vi "BoxBegin.vi"   [LabVIEW 2023]
uses:
  <vilib>/Rock Robotics/WPI/ThirdParty/REV Robotics/REVLib/Typedef/Spark MAX Idle Mode.ctl
  <vilib>/Rock Robotics/WPI/ThirdParty/REV Robotics/REVLib/Typedef/Spark MAX Sensor Type.ctl
  <vilib>/Rock Robotics/WPI/ThirdParty/REV Robotics/REVLib/Typedef/Spark MAX Motor Type.ctl
types:
  T1 = typedef "Spark MAX Sensor Type.ctl" = enum16{"No Sensor", "Hall Sensor", "Encoder", "-Not Available-", "Analog", "Alternate Encoder", "Duty Cycle"}
  T2 = typedef "Spark MAX Idle Mode.ctl" = enum16{"Coast", "Brake"}
  T3 = typedef "Spark MAX Motor Type.ctl" = enum16{"Brushed", "Brushless"}
  T4 = typedef "WPI_MotorControlDeviceRef.ctl" = cluster{"DeviceStatus":errorcluster, "Type":T5, "PWM":cluster{"PWM Channel":T6, "DeadBand":T7}, "CAN":cluster{"Device Number":u8, "SetOutput VI Ref":variant, "GetOutput VI Ref":variant, "Enable VI Ref":variant, "Disable VI Ref":variant, "Data":variant}, "Invert":bool, "DIO PWM":cluster{"PWM \"Enable\" Channel":T6, "DIOChannel":T8, "PWM Rate":dbl}}
  T5 = typedef "WPI_MotorControlType.ctl" = enum16{"PWM", "CAN", "DIO PWM"}
  T6 = typedef "FPGA_DIOPWMChannel.ctl" = enum8{"PWM 0", "PWM 1", "PWM 2", "PWM 3", "PWM 4", "PWM 5", "PWM 6", "PWM 7", "PWM 8", "PWM 9", "PWM MXP 0", "PWM MXP 1", "PWM MXP 2", "PWM MXP 3", "PWM MXP 4", "PWM MXP 5", "PWM MXP 6", "PWM MXP 7", "PWM MXP 8", "PWM MXP 9", "Invalid"}
  T7 = typedef "WPI_PWMDeadband.ctl" = cluster{"Name":string, "maxPositivePwm":i32, "minPositivePwm":i32, "centerPwm":i32, "maxNegativePwm":i32, "minNegativePwm":i32, "angularRange":u16}
  T8 = typedef "FPGA_DIOChannel.ctl" = enum8{"DIO 0", "DIO 1", "DIO 2", "DIO 3", "DIO 4", "DIO 5", "DIO 6", "DIO 7", "DIO 8", "DIO 9", "DIO MXP 0", "DIO MXP 1", "DIO MXP 2", "DIO MXP 3", "DIO MXP 4", "DIO MXP 5", "DIO MXP 6", "DIO MXP 7", "DIO MXP 8", "DIO MXP 9", "DIO MXP 10", "DIO MXP 11", "DIO MXP 12", "DIO MXP 13", "DIO MXP 14", "DIO MXP 15", "SPI Port CS1", "SPI Port CS2", "SPI Port CS3", "SPI Port MISO", "SPI Port MOSI", "Invalid"}
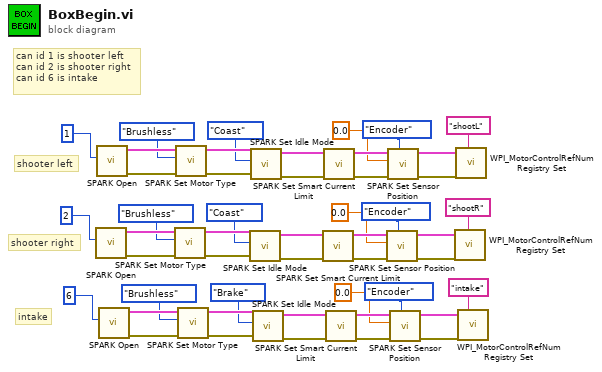
[diagram p0: block diagram]
diagram:
  # "intake"
  # "shooter right"
  # "shooter left"
  # "can id 1 is shooter left\ncan id 2 is shooter right\ncan id 6 is intake"
  n1 = call <vilib>:"SPARK Open.vi"("Device Number"=2) -> ("error out"=w25:errorcluster, "MotorControlDeviceRef"=w29:T4)  [unwired: 9 in]
  n2 = call <vilib>:"SPARK Open.vi"("Device Number"=1) -> ("error out"=w41:errorcluster, "MotorControlDeviceRef"=w45:T4)  [unwired: 9 in]
  n3 = call <vilib>:"SPARK Open.vi"("Device Number"=6) -> ("error out"=w9:errorcluster, "MotorControlDeviceRef"=w13:T4)  [unwired: 9 in]
  n4 = call <vilib>:"SPARK Set Motor Type.vi"("error in (no error)"=w25, "Motor Type"=Spark_MAX_Motor_Type."Brushless", "MotorControlDevRef"=w29) -> ("error out"=w24:errorcluster, "MotorControlDeviceRef"=w28:T4)  [unwired: 7 in]
  n5 = call <vilib>:"SPARK Set Motor Type.vi"("error in (no error)"=w41, "Motor Type"=Spark_MAX_Motor_Type."Brushless", "MotorControlDevRef"=w45) -> ("error out"=w40:errorcluster, "MotorControlDeviceRef"=w44:T4)  [unwired: 7 in]
  n6 = call <vilib>:"SPARK Set Motor Type.vi"("error in (no error)"=w9, "Motor Type"=Spark_MAX_Motor_Type."Brushless", "MotorControlDevRef"=w13) -> ("error out"=w8:errorcluster, "MotorControlDeviceRef"=w12:T4)  [unwired: 7 in]
  n7 = call <vilib>:"SPARK Set Idle Mode.vi"("error in (no error)"=w24, "Idle Mode"=Spark_MAX_Idle_Mode."Coast", "MotorControlDeviceRef in"=w28) -> ("error out"=w23:errorcluster, "MotorControlDeviceRef out"=w27:T4)  [unwired: 7 in]
  n8 = call <vilib>:"SPARK Set Idle Mode.vi"("error in (no error)"=w40, "Idle Mode"=Spark_MAX_Idle_Mode."Coast", "MotorControlDeviceRef in"=w44) -> ("error out"=w39:errorcluster, "MotorControlDeviceRef out"=w43:T4)  [unwired: 7 in]
  n9 = call <vilib>:"SPARK Set Idle Mode.vi"("error in (no error)"=w8, "Idle Mode"=Spark_MAX_Idle_Mode."Brake", "MotorControlDeviceRef in"=w12) -> ("error out"=w7:errorcluster, "MotorControlDeviceRef out"=w11:T4)  [unwired: 7 in]
  n10 = call <vilib>:"SPARK Set Smart Current Limit.vi"("error in (no error)"=w23, "MotorControlDeviceRef in"=w27) -> ("error out"=w22:errorcluster, "MotorControlDeviceRef out"=w26:T4)  [unwired: 8 in]
  n11 = call <vilib>:"SPARK Set Smart Current Limit.vi"("error in (no error)"=w39, "MotorControlDeviceRef in"=w43) -> ("error out"=w38:errorcluster, "MotorControlDeviceRef out"=w42:T4)  [unwired: 8 in]
  n12 = call <vilib>:"SPARK Set Smart Current Limit.vi"("error in (no error)"=w7, "MotorControlDeviceRef in"=w11) -> ("error out"=w6:errorcluster, "MotorControlDeviceRef out"=w10:T4)  [unwired: 8 in]
  n13 = call <vilib>:"SPARK Set Sensor Position.vi"("Sensor Type (Hall Sensor)"=Spark_MAX_Sensor_Type."Encoder", "error in"=w22, "Position"=0.0, "MotorControlDeviceRef"=w26) -> ("error out"=w21:errorcluster, "MotorControlDeviceRef"=w30:T4)  [unwired: 6 in]
  n14 = call <vilib>:"SPARK Set Sensor Position.vi"("Sensor Type (Hall Sensor)"=Spark_MAX_Sensor_Type."Encoder", "error in"=w38, "Position"=0.0, "MotorControlDeviceRef"=w42) -> ("error out"=w37:errorcluster, "MotorControlDeviceRef"=w46:T4)  [unwired: 6 in]
  n15 = call <vilib>:"SPARK Set Sensor Position.vi"("Sensor Type (Hall Sensor)"=Spark_MAX_Sensor_Type."Encoder", "error in"=w6, "Position"=0.0, "MotorControlDeviceRef"=w10) -> ("error out"=w5:errorcluster, "MotorControlDeviceRef"=w14:T4)  [unwired: 6 in]
  n16 = call <vilib>:"WPI_MotorControlRefNum Registry Set.vi"("error in (no error)"=w21, "refnum name"="shootR", "MotorControlDevRef"=w30) -> ()  [unwired: 7 in, 2 out]
  n17 = call <vilib>:"WPI_MotorControlRefNum Registry Set.vi"("error in (no error)"=w37, "refnum name"="shootL", "MotorControlDevRef"=w46) -> ()  [unwired: 7 in, 2 out]
  n18 = call <vilib>:"WPI_MotorControlRefNum Registry Set.vi"("error in (no error)"=w5, "refnum name"="intake", "MotorControlDevRef"=w14) -> ()  [unwired: 7 in, 2 out]
